vi "MHM Write Register.vi"(7 "pulData":u32[](array[numeric]), 8 "error in (no error)":errorcluster, 9 "pulNumberOfBytes":u32, 10 "ulAdr":u32, 11 "ulMHMHandle":u32) -> (0 "error out":errorcluster, 2 "pulNumberOfBytes out":u32, 3 "function return":u32)   [LabVIEW 2017, in "MHM_1SL_interface.lvlib"]
uses:
  MHM_1SL_interface.lvlib
  SSI_Tool/DUT_Interface/lv_interface/lib/MHM_1SL_interface.dll
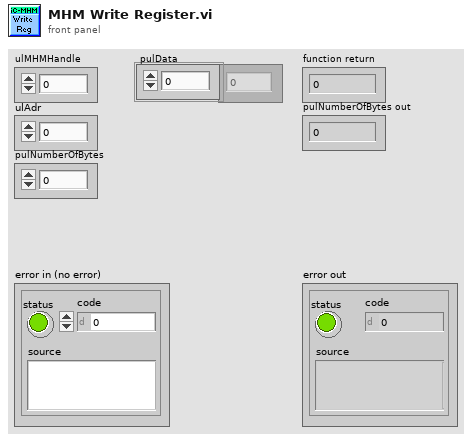
[diagram p1: front panel]
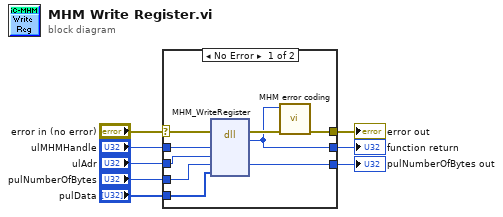
[diagram p0: block diagram]
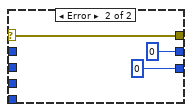
[diagram p2: hidden frame]
diagram:
  n1 = case shown="No Error" "error in (no error)" {
    selector: "error in (no error)" -> [w17 w20]
    tunnel: "ulMHMHandle" -> [w16 _]
    tunnel: [w14 w20] -> w6
    tunnel: [w13 u32 0 ("return type")] -> w5
    tunnel: "ulAdr" -> [w12 _]
    tunnel: "pulNumberOfBytes" -> [w11 _]
    tunnel: [w10 u32 0 ("return type")] -> w2
    tunnel: "pulData" -> [w9 _]
    frame No Error {
      n2 = dll-call lib="C:/workspace/project/scancon/sw/SSI_Tool/DUT_Interface/lv_interface/lib/MHM_1SL_interface.dll" fn="MHM_WriteRegister"(error in=w17, "ulMHMHandle"=w16, "ulAdr"=w12, "pulNumberOfBytes"=w11, "pulData"=w9) -> (error out=w15:errorcluster, "return type"=w13:u32, "pulNumberOfBytes"=w10:u32)  [unwired: 5 in, 1 out]
      n3 = call "MHM error coding.vi"("error in (no error)"=w15, "function return in"=w13) -> ("error out"=w14:errorcluster)  [unwired: 9 in]
    }
    frame Error {
    }
  }
  "function return" <- w5
  "error out" <- w6
  "pulNumberOfBytes out" <- w2
